vi "Read Dev Mode.vi"(8 "error in (no error)":errorcluster, 11 "VISA resource name":refnum<visa-resource-name>) -> (0 "error out":errorcluster, 2 "dev mode":bool, 3 "VISA resource name out":refnum<visa-resource-name>)   [LabVIEW 2019, in "Andeen-Hagerling 2700A.lvlib"]
doc: "Returns a boolean indicating whether or not the deviation mode i\nis enabled.\n\nWhen enabled, the deviation mode takes capacitance and \nloss measurements very rapidly and converts them to analog\nvoltages that are proportional to the measured capacitance \nand loss. This is a special mode of operation that functions as\na high-speed alternative to the normal bridge mode measurements."
uses:
  Andeen-Hagerling 2700A.lvlib
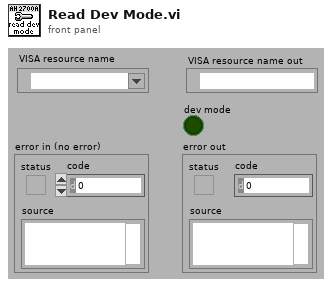
[diagram p1: front panel]
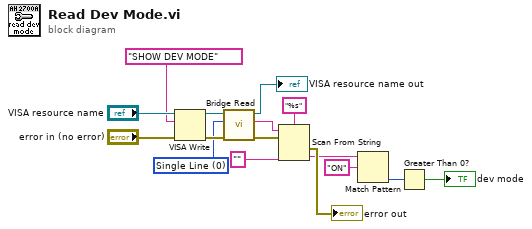
[diagram p0: block diagram]
diagram:
  w1 = u16 0 items=["Single Line", "Multi-Line"] ("Multiline")
  n1 = VISA Write(VISA resource name="VISA resource name", write buffer="SHOW DEV MODE" ("command"), error in (no error)="error in (no error)") -> (VISA resource name out=w3:refnum<visa-resource-name>, error out=w2:errorcluster)  [unwired: 1 out]
  n2 = call "Bridge Read.vi"("error in (no error)"=w2, "multiline"=w1, "VISA resource name"=w3) -> ("error out"=w5:errorcluster, "read buffer"=w6:string, "VISA resource name out"=→"VISA resource name out":refnum<visa-resource-name>)  [unwired: 6 in]
  n3 = Scan From String(format string="%s", input string=w6, error in=w5, default 1="" ("default value 1")) -> (error out=→"error out":errorcluster, output 1=w11:string)  [unwired: 1 in, 2 out]
  n4 = Match Pattern(string=w11, regular expression="ON") -> (offset past match=w8:i32)  [unwired: 1 in, 3 out]
  n5 = Greater Than 0?(x=w8) -> (x > 0?=→"dev mode":bool)
